vi "test1.vi"() -> ()   [LabVIEW 2016]
uses:
  <vilib>/Instr/_visa.llb/VISA Configure Serial Port (Instr).vi
panel:
  in  "DTR Write":bool
  in  "RTS Write":bool
  out "return count":u32
  in  "write buffer":string
  in  "send":bool
  in  "stop":bool
  in  "VISA resource name":refnum<visa-resource-name>
  # "1 - адресс 1 двигателя\n2 - адресс 2 двигателя\n$0MV\\01+   - запуск всех двигателей в положительном направлении \n$0MS\\00   - остановка всех двигателей\n$0MJ\\04+\\00\\00\\01   - 1 шаг всех двигателей\n$0SS\\01\\10   - скорость 10 для всех двигателей"
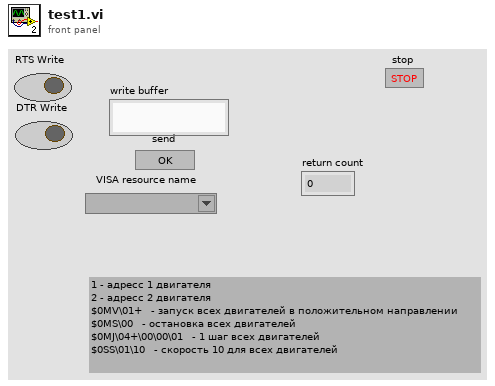
[diagram p1: front panel]
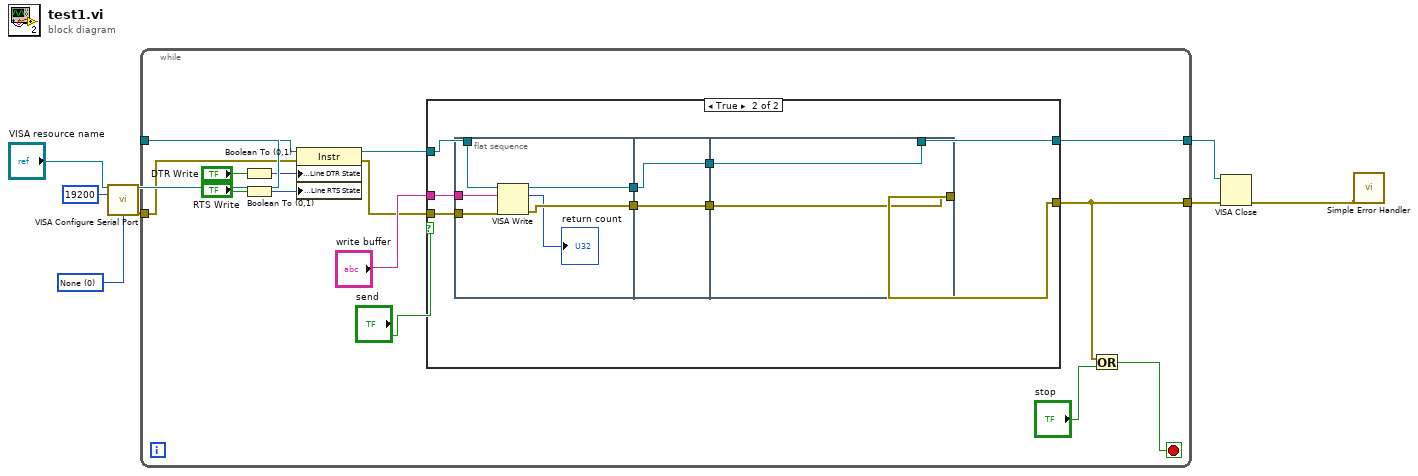
[diagram p0: block diagram]
diagram:
  w1 = u16 0 items=["None", "XON/XOFF", "RTS/CTS", "XON/XOFF & RTS/CTS", "DTR/DSR", "XON/XOFF & DTR/DSR"] ("flow control (0:none)")
  n1 = call-poly "VISA Configure Serial Port"("VISA resource name"="VISA resource name", "baud rate (9600)"=u32 19200, "flow control (0:none)"=w1) -> ("VISA resource name out"=w4:refnum<visa-resource-name>, "error out"=w5:errorcluster)  [unwired: 11 in]
  n2 = while {
    tunnel: w5 -> [w11]
    tunnel: [w19] -> w8
    tunnel: w4 -> [w12]
    tunnel: [w20] -> w7
    stop <- w22 stop-if-true
    n3 = Boolean To (0,1)(Boolean="DTR Write") -> (0, 1=w16:i16)
    n4 = Boolean To (0,1)(Boolean="RTS Write") -> (0, 1=w14:i16)
    n5 = property class="Instr"(reference=w12, error in=w11, "Serial Settings:Modem Line Settings:Line DTR State"=w16, "Serial Settings:Modem Line Settings:Line RTS State"=w14) -> (reference out=w9:refnum<visa-resource-name>, error out=w10:errorcluster)
    n6 = case shown="True" "send" {
      tunnel: [w24 w26] -> w19
      tunnel: [w23 w27] -> w20
      tunnel: "write buffer" -> [_ w33]
      tunnel: w10 -> [w24 w32]
      tunnel: w9 -> [w23 w25]
      frame False {
      }
      frame True {
        n7 = flat-sequence {
          tunnel: w33 -> [w39]
          tunnel: w32 -> [w38]
          tunnel: w25 -> [w37]
          tunnel: [w36] -> w30
          tunnel: [w35] -> w28
          tunnel: [w41] -> w31
          tunnel: w30 -> [w41]
          tunnel: [w40] -> w29
          tunnel: w28 -> [w40]
          tunnel: w31 -> [w43]
          tunnel: w29 -> [w42]
          tunnel: [w43] -> w27
          tunnel: [w42] -> w26
          frame #0 {
            n8 = VISA Write(VISA resource name=w37, write buffer=w39, error in (no error)=w38) -> (VISA resource name out=w36:refnum<visa-resource-name>, return count=→"return count":u32, error out=w35:errorcluster)
          }
          frame #1 {
          }
          frame #2 {
          }
        }
      }
    }
    n9 = Or(x=w19, y="stop") -> (x .or. y?=w22:bool)
  }
  n10 = VISA Close(VISA resource name=w7, error in (no error)=w8) -> (error out=w6:errorcluster)
  n11 = call <vilib>:"Simple Error Handler.vi"("error in (no error)"=w6) -> ()  [unwired: 4 in, 5 out]
